vi "WAPIAerReadStatus-SingleAxe.vi"(3 "nAxis":i16(ring)=1 items=["Axis 1"=1, "Axis 2"=2, "Axis 3"=3, "Axis 4"=4], 9 "error in (no error)":errorcluster) -> (0 "Axis status":T1, 6 "error out":errorcluster)   [LabVIEW 2009]
uses:
  win50032.dll
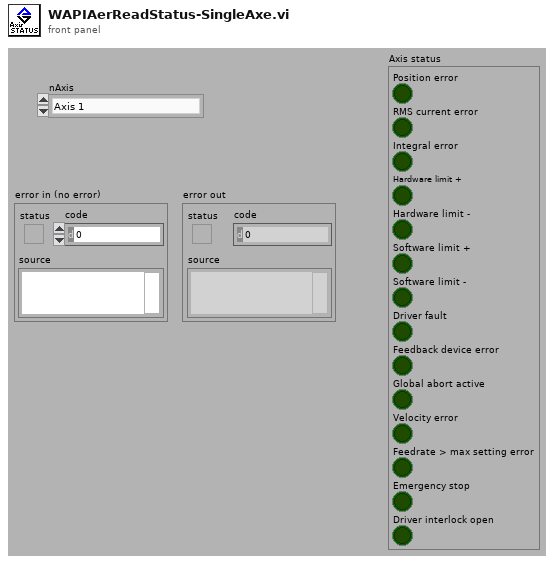
[diagram p1: front panel]
types:
  T1 = cluster{"Position error":bool, "RMS current error":bool, "Integral error":bool, "Hardware limit +":bool, "Hardware limit -":bool, "Software limit +":bool, "Software limit -":bool, "Driver fault":bool, "Feedback device error":bool, "Global abort active":bool, "Velocity error":bool, "Feedrate > max setting error":bool, "Emergency stop":bool, "Driver interlock open":bool}
  T2 = cluster{"Boolean array[0]":bool, "Boolean array[1]":bool, "Boolean array[2]":bool, "Boolean array[3]":bool, "Boolean array[4]":bool, "Boolean array[5]":bool, "Boolean array[6]":bool, "Boolean array[7]":bool, "Boolean array[8]":bool, "Boolean array[9]":bool, "Boolean array[10]":bool, "Boolean array[11]":bool, "Boolean array[12]":bool, "Boolean array[13]":bool}
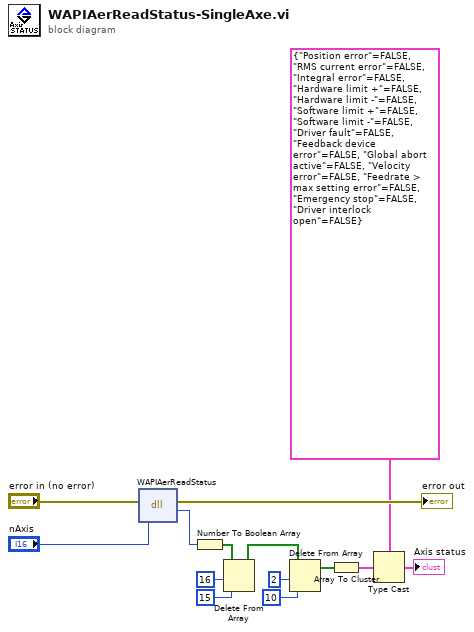
[diagram p0: block diagram]
diagram:
  n1 = dll-call lib="win50032.dll" fn="WAPIAerReadStatus"(error in="error in (no error)", "nStatus"="nAxis") -> (error out=→"error out":errorcluster, "return type"=w11:u32)  [unwired: 3 in, 1 out]
  n2 = Number To Boolean Array(number=w11) -> (Boolean array=w8:bool[])
  n3 = Delete From Array(array=w8, length=16, index=15) -> (array with subset deleted=w7:bool[])  [unwired: 1 out]
  n4 = Delete From Array(array=w7, length=2, index=10) -> (array with subset deleted=w4:bool[])  [unwired: 1 out]
  n5 = Array To Cluster(array=w4) -> (cluster=w3:T2)
  n6 = Type Cast(type=T1 {"Position error"=FALSE, "RMS current error"=FALSE, "Integral error"=FALSE, "Hardware limit +"=FALSE, "Hardware limit -"=FALSE, "Software limit +"=FALSE, "Software limit -"=FALSE, "Driver fault"=FALSE, "Feedback device error"=FALSE, "Global abort active"=FALSE, "Velocity error"=FALSE, "Feedrate > max setting error"=FALSE, "Emergency stop"=FALSE, "Driver interlock open"=FALSE}, x=w3) -> (*(type *) &x=→"Axis status":T1)
